vi "updateHighScore.vi"(8 "error in (no error)":errorcluster, 11 "Player in":refnum<class "Player.lvclass">) -> (0 "error out":errorcluster, 2 "High Score Updated?":bool, 3 "Player out":refnum<class "Player.lvclass">)   [LabVIEW 2020, in "Player.lvclass"]
uses:
  Player.lvclass
  Player.lvclass/Player.ctl
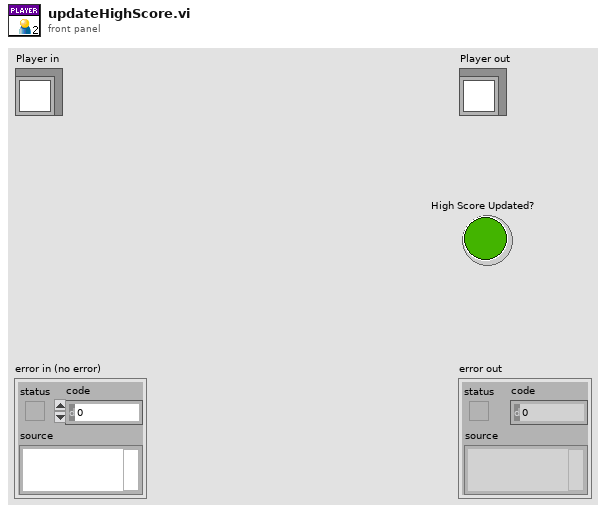
[diagram p1: front panel]
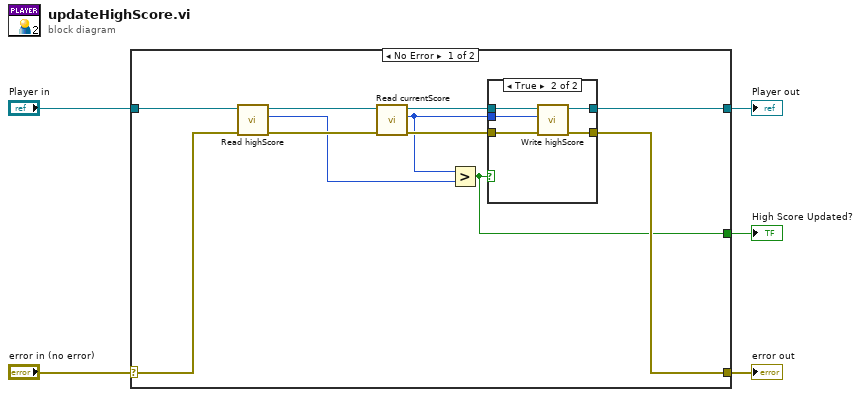
[diagram p0: block diagram]
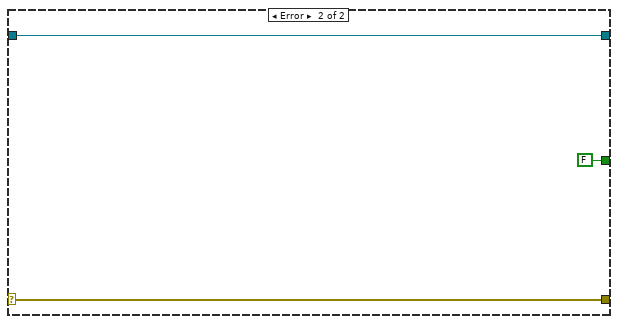
[diagram p3: hidden frame]
diagram:
  n1 = case shown="No Error" "error in (no error)" {
    selector: "error in (no error)" -> [w16 w26]
    tunnel: [w11 w26] -> w4
    tunnel: [w9 w25] -> w2
    tunnel: "Player in" -> [w14 w25]
    tunnel: [w7 FALSE] -> w1
    frame No Error {
      n2 = call "Read highScore.vi"("error in (no error)"=w16, "Player in"=w14) -> ("error out"=w15:errorcluster, "highScore"=w8:u64, "Player out"=w12:refnum<class "Player.lvclass">)  [unwired: 7 in]
      n3 = call "Read currentScore.vi"("error in (no error)"=w15, "Player in"=w12) -> ("error out"=w13:errorcluster, "currentScore"=w6:u64, "Player out"=w10:refnum<class "Player.lvclass">)  [unwired: 7 in]
      n4 = Greater?(x=w6, y=w8) -> (0:w7:bool)
      n5 = case shown="True" w7 {
        tunnel: w13 -> [w17 w23]
        tunnel: [w17 w22] -> w11
        tunnel: w10 -> [w18 w21]
        tunnel: [w18 w20] -> w9
        tunnel: w6 -> [_ w19]
        frame False {
        }
        frame True {
          n6 = call "Write highScore.vi"("error in (no error)"=w23, "highScore"=w19, "Player in"=w21) -> ("error out"=w22:errorcluster, "Player out"=w20:refnum<class "Player.lvclass">)  [unwired: 7 in]
        }
      }
    }
    frame Error {
    }
  }
  "error out" <- w4
  "Player out" <- w2
  "High Score Updated?" <- w1
